vi "Commands.vi"(8 "error in (no error)":errorcluster, 11 "VISA resource name":refnum<visa-resource-name>) -> (0 "error out":errorcluster, 2 "Commands":string, 3 "VISA resource name out":refnum<visa-resource-name>)   [LabVIEW 2017, in "RadWag balances and scales.lvlib"]
doc: "Returns all comands suported by balance."
uses:
  <instrlib>/Radwag Balances and Scales/Public/RadWag balances and scales.lvlib
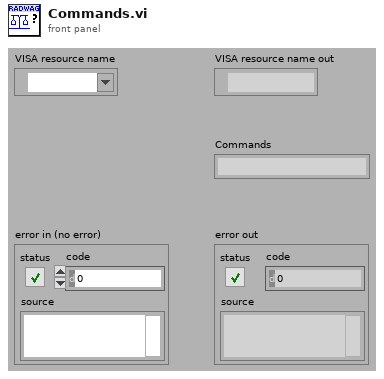
[diagram p1: front panel]
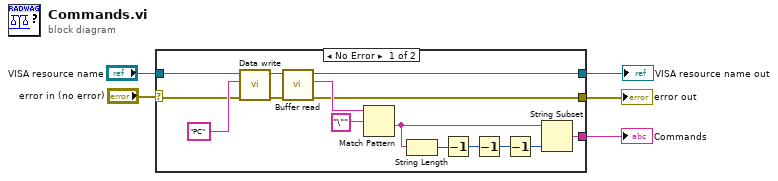
[diagram p0: block diagram]
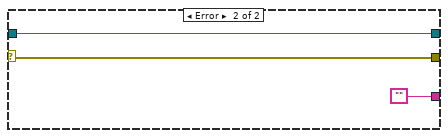
[diagram p2: hidden frame]
diagram:
  n1 = case shown="No Error" "error in (no error)" {
    selector: "error in (no error)" -> [w7 w22]
    tunnel: [w6 w23] -> w1
    tunnel: [w10 ""] -> w4
    tunnel: [w9 w22] -> w3
    tunnel: "VISA resource name" -> [w8 w23]
    frame No Error {
      n2 = call <instrlib>:"Data write.vi"("error in (no error)"=w7, "ID"="PC", "VISA resource name"=w8) -> ("error out"=w18:errorcluster, "VISA resource name out"=w19:refnum<visa-resource-name>)  [unwired: 7 in]
      n3 = call <instrlib>:"Buffer read.vi"("error in (no error)"=w18, "VISA resource name"=w19) -> ("error out"=w9:errorcluster, "Received String"=w17:string, "VISA resource name out"=w6:refnum<visa-resource-name>)  [unwired: 7 in]
      n4 = Match Pattern(string=w17, regular expression="\"") -> (after substring=w14:string)  [unwired: 1 in, 3 out]
      n5 = String Length(string=w14) -> (length=w15:i32)
      n6 = Decrement(x=w15) -> (x-1=w12:i32)
      n7 = Decrement(x=w12) -> (x-1=w11:i32)
      n8 = Decrement(x=w11) -> (x-1=w13:i32)
      n9 = String Subset(string=w14, length (rest)=w13) -> (substring=w10:string)  [unwired: 1 in]
    }
    frame Error {
    }
  }
  "Commands" <- w4
  "error out" <- w3
  "VISA resource name out" <- w1
